vi "Remove Error.vi"(7 "scope":T1=enum."global", 8 "error in (no error)":errorcluster, 10 "selected error":T2, 11 "error list <top> in":variant) -> (0 "error out":errorcluster, 3 "error list <top> out":variant)   [LabVIEW 2017]
uses:
  Error Owner and ID.ctl
  Scope.ctl
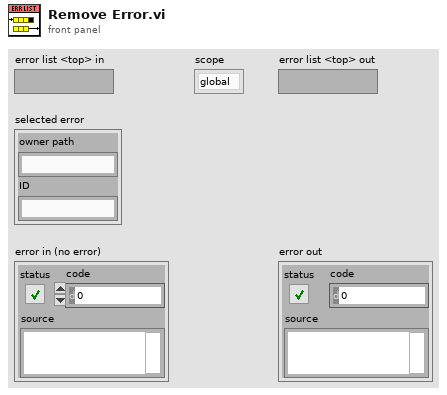
[diagram p1: front panel]
types:
  T1 = typedef "Scope.ctl" = enum16{"project", "global"}
  T2 = typedef "Error Owner and ID.ctl" = cluster{"owner path":string, "ID":string}
  T3 = typedef "Error Code File Properties.ctl" = cluster{"path":path, "simplified path":string, "name":string, "display name":string, "family name":string, "comment":string, "parsable?":bool, "file modified?":bool}
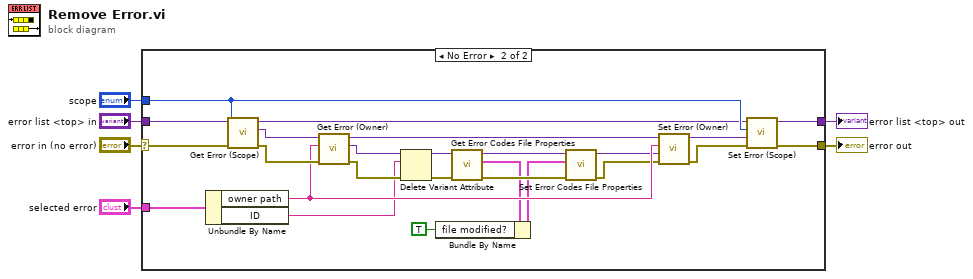
[diagram p0: block diagram]
diagram:
  n1 = case shown="No Error" "error in (no error)" {
    selector: "error in (no error)" -> [w8 w19]
    tunnel: "scope" -> [_ w32]
    tunnel: "selected error" -> [_ w23]
    tunnel: [w8 w20] -> w3
    tunnel: "error list <top> in" -> [w7 w18]
    tunnel: [w7 w17] -> w1
    frame Error {
    }
    frame No Error {
      n2 = Unbundle By Name(w23) -> ("owner path"=w22:string, "ID"=w21:string)
      n3 = call "Get Error (Scope).vi"("error in (no error)"=w19, "scope"=w32, "error list <top>"=w18) -> ("error out"=w29:errorcluster, "error list <scope>"=w28:variant, "error list <top> dup"=w27:variant)  [unwired: 5 in, 1 out]
      n4 = call "Get Error (Owner).vi"("error in (no error)"=w29, "owner"=w22, "error list <scope>"=w28) -> ("error out"=w25:errorcluster, "error list <owner>"=w24:variant, "error list <scope> dup"=w26:variant)  [unwired: 5 in, 1 out]
      n5 = Delete Variant Attribute(4:w25, 6:w21, 7:w24) -> (0:w15:errorcluster, 3:w16:variant)  [unwired: 1 out]
      n6 = call "Get Error Codes File Properties.vi"("error in (no error)"=w15, "error list <owner> in"=w16) -> ("error out"=w33:errorcluster, "properties"=w11:T3, "error list <owner> out"=w14:variant)  [unwired: 6 in, 1 out]
      n7 = Bundle By Name(cluster=w11, "file modified?"=TRUE) -> (w10:T3)
      n8 = call "Set Error Codes File Properties.vi"("error in (no error)"=w33, "properties"=w10, "error list <owner> in"=w14) -> ("error out"=w12:errorcluster, "error list <owner> out"=w13:variant)  [unwired: 7 in]
      n9 = call "Set Error (Owner).vi"("error in (no error)"=w12, "error list <owner>"=w13, "owner"=w22, "error list <scope> in"=w26) -> ("error out"=w30:errorcluster, "error list <scope> out"=w31:variant)  [unwired: 6 in]
      n10 = call "Set Error (Scope).vi"("error in (no error)"=w30, "error list <scope>"=w31, "scope"=w32, "error list <top> in"=w27) -> ("error out"=w20:errorcluster, "error list <top> out"=w17:variant)  [unwired: 6 in]
    }
  }
  "error out" <- w3
  "error list <top> out" <- w1
